vi "get_current_repetition.vi"(8 "error in (no error)":errorcluster, 11 "DL090211ImageAssemblerScaffold.lvclass in":refnum<class "ImageAssemblerDL090211Scaffold.lvclass">) -> (0 "error out":errorcluster, 2 "current repetition":i32=1, 3 "DL090211ImageAssemblerScaffold.lvclass out":refnum<class "ImageAssemblerDL090211Scaffold.lvclass">)   [LabVIEW 2010, in "ImageAssemblerDL090211Scaffold.lvclass"]
uses:
  ImageAssemblerDL090211Scaffold.lvclass
  ImageAssemblerDL090211Scaffold.lvclass/ImageAssemblerDL090211Scaffold.ctl
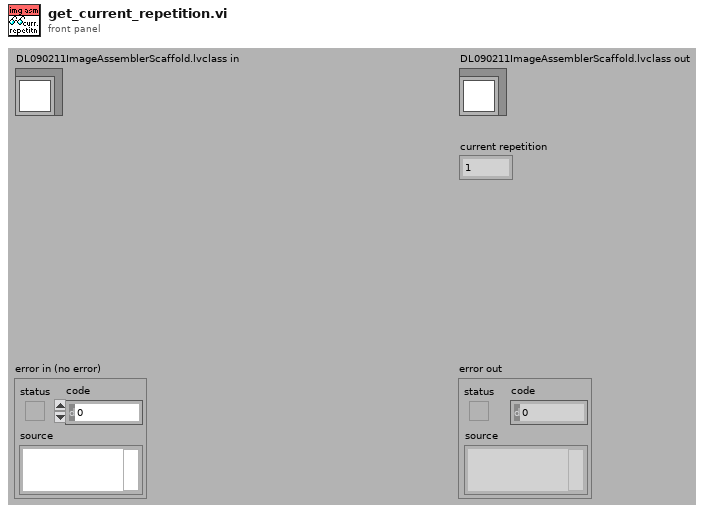
[diagram p1: front panel]
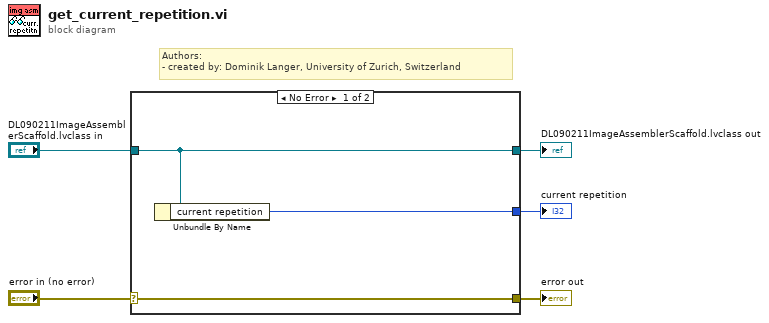
[diagram p0: block diagram]
diagram:
  # "Authors: \n- created by: Dominik Langer, University of Zurich, Switzerland"
  n1 = case shown="No Error" "error in (no error)" {
    selector: "error in (no error)" -> [w8 w9]
    tunnel: [w8 w9] -> w4
    tunnel: [w7 w10] -> w2
    tunnel: "DL090211ImageAssemblerScaffold.lvclass in" -> [w7 w10]
    tunnel: [w6 _] -> w1
    frame No Error {
      n2 = Unbundle By Name(w7) -> ("current repetition"=w6:i32)
    }
    frame Error {
    }
  }
  "error out" <- w4
  "DL090211ImageAssemblerScaffold.lvclass out" <- w2
  "current repetition" <- w1
